vi "Do.vi"(8 "error in":errorcluster, 10 "Actor in":refnum<class "Actor.lvclass">, 11 "Send CRD Data":refnum<class "Send CRD Data.lvclass">) -> (0 "error out":errorcluster, 2 "Actor out":refnum<class "Actor.lvclass">)   [LabVIEW 2014, in "Send CRD Data.lvclass"]
doc: "(<B>Filename</B>: Actor Framework.lvlib:Message.lvclass:Do.vi)\n\nDefines what a message does when it is received by an actor. Generally, a message instructs an actor to invoke one of its methods. By default, this method does nothing. A child class must override it to define behavior. Create a child class by using the Actor Framework Message Maker dialog box."
uses:
  Send CRD Data.lvclass
  <vilib>/ActorFramework/Actor/Actor.lvclass
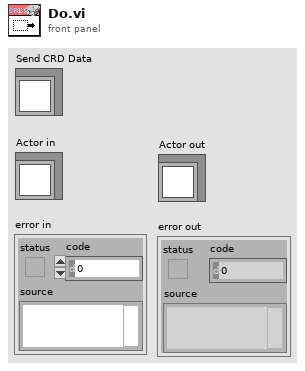
[diagram p1: front panel]
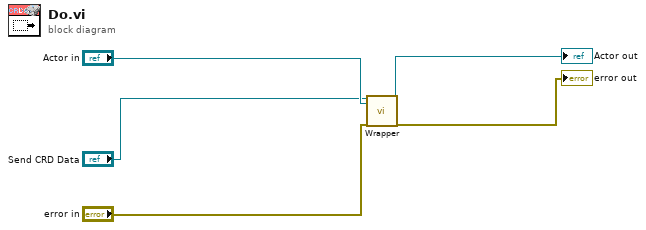
[diagram p0: block diagram]
diagram:
  n1 = call "Wrapper.vi"("Send CRD Data in"="Send CRD Data", "Actor in"="Actor in", "error in (no error)"="error in") -> ("Controller out"=→"Actor out":refnum<class "Controller.lvclass">, "error out"=→"error out":errorcluster)  [unwired: 15 in]
